vi "GenerateEventLog.vi"(0 "Instrument":string="Control", 2 "Check for file?":bool=TRUE) -> (3 "Global File Information":T1, 5 "File Path Out":path=path "D:/Data/2018-06-15/Proj_1/Temp Dependence/Control_200C.tdms")   [LabVIEW 2018]
uses:
  Global Variables.vi
  <vilib>/Utility/file.llb/Read Delimited Spreadsheet (string).vi
panel:
  in  "Path":path=path "E:/ProjectIndex.csv"
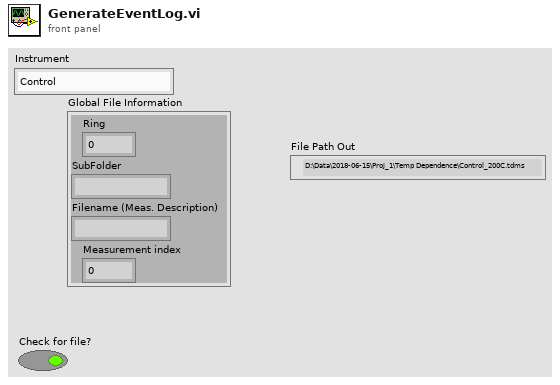
[diagram p1: front panel]
types:
  T1 = cluster{"Ring":u16, "SubFolder":string, "Filename (Meas. Description)":string, "Measurement index":i32}
  T2 = cluster{"Project":u16, "SubFolder":string, "Filename (Meas. Description)":string, "Measurement index":i32}
  T3 = cluster{"Project":u16, "SubFolder 2":string, "Meas. Description 2":string, "Measurement number 2":i32}
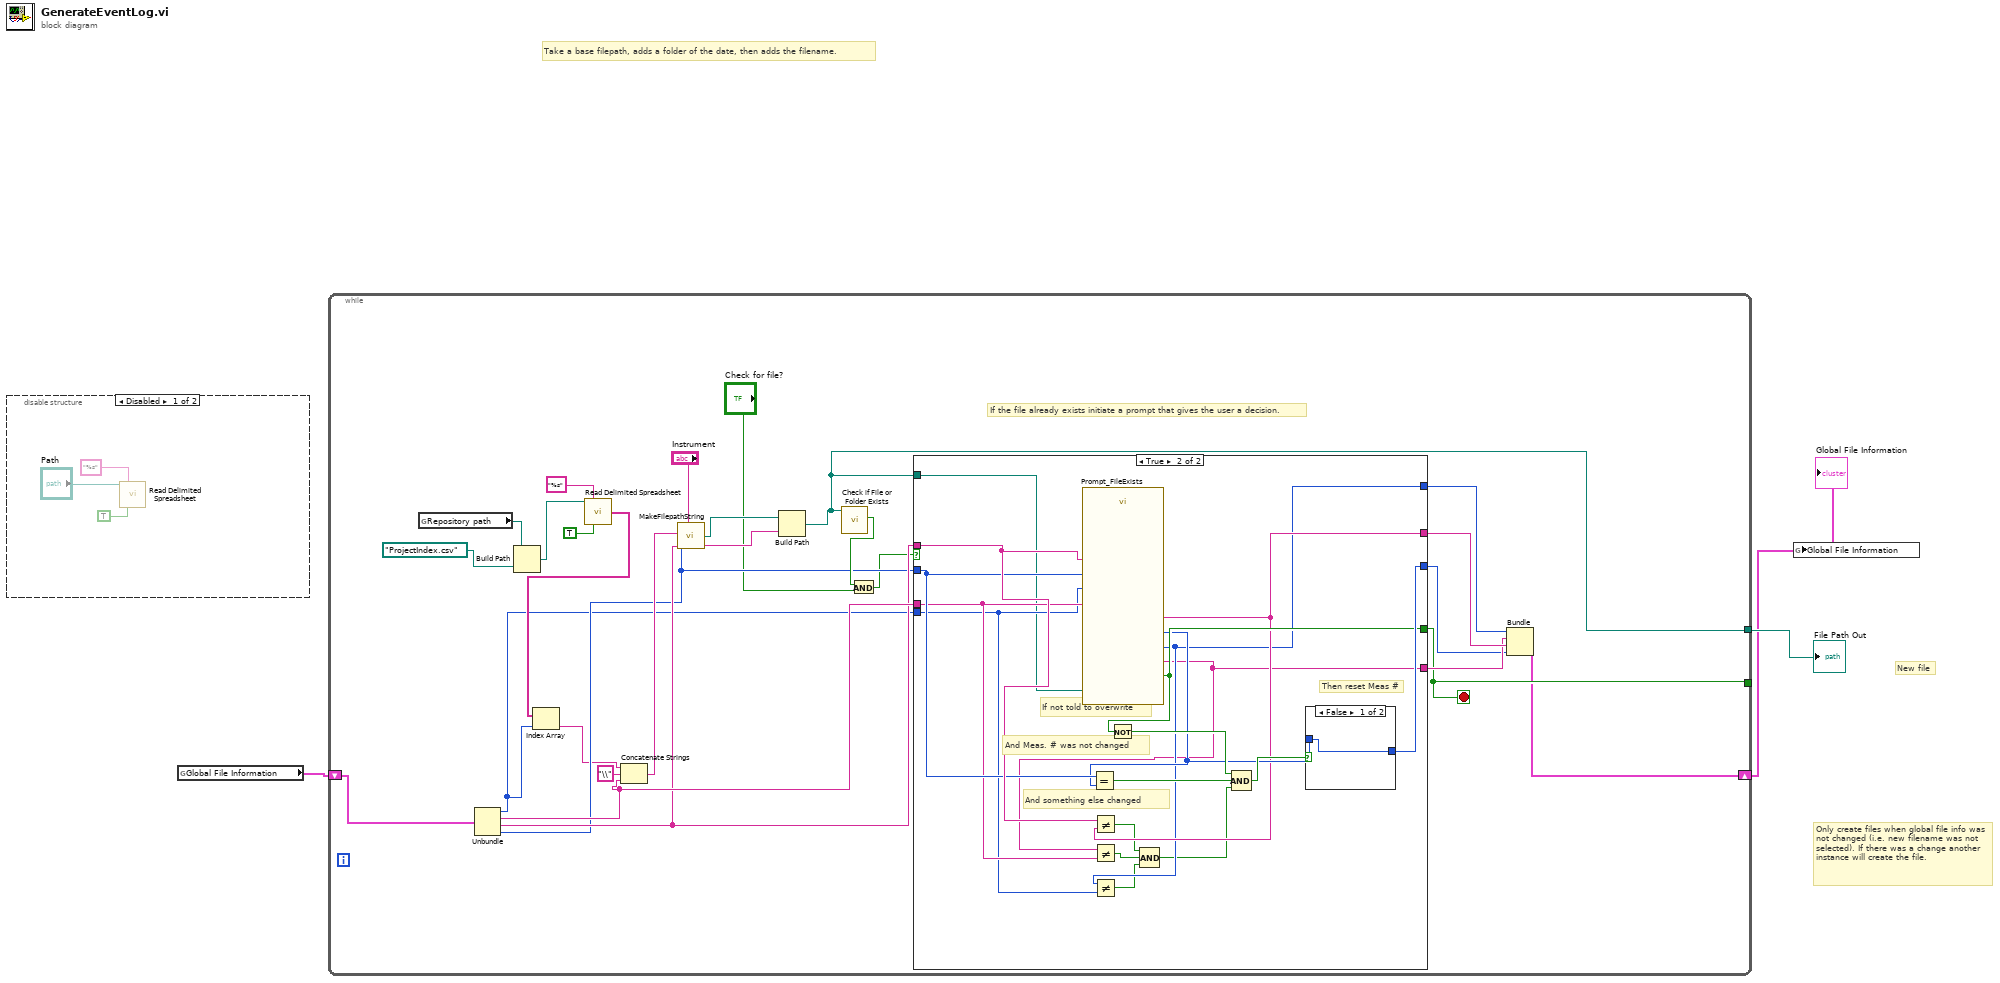
[diagram p0: block diagram]
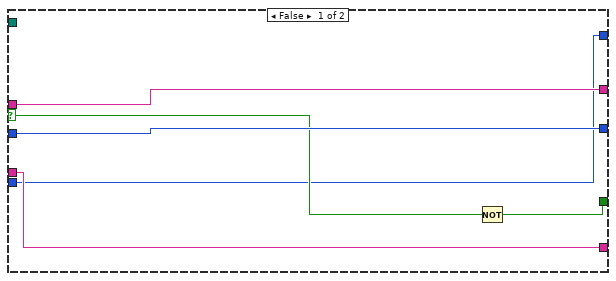
[diagram p3: hidden frame]
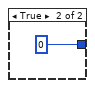
[diagram p4: hidden frame]
diagram:
  # "Only create files when global file info was not changed (i.e. new filename was not selected). If there was a change another instance will create the file."
  # "New file"
  # "Take a base filepath, adds a folder of the date, then adds the filename."
  n1 = disable-structure shown="Disabled" {
    frame Disabled {
      n2 = call-poly <vilib>:"Read Delimited Spreadsheet.vi"("file path (dialog if empty)"="Path", "format (%s)"="%s", "transpose? (F)"=TRUE) -> ("first row"=w4:string[])  [unwired: 7 in, 5 out]
    }
    frame Enabled {
    }
  }
  n3 = global read "Global Variables.vi" "Global File Information"() -> (w2:T2)
  n4 = while {
    tunnel: [w20] -> w3
    tunnel: [w19] -> _
    shift-right: [w17] -> w1
    shift-left: w2 -> [w16]
    stop <- w19 stop-if-true
    # "If the file already exists initiate a prompt that gives the user a decision."
    n5 = global read "Global Variables.vi" "Repository path"() -> (w15:path)
    n6 = Unbundle(w16) -> ("Project"=w9:u16, "SubFolder"=w29:string, "Filename (Meas. Description)"=w28:string, "Measurement index"=w27:i32)
    n7 = Build Path(base path=w15, name or relative path=path "ProjectIndex.csv" ("vi path")) -> (appended path=w14:path)
    n8 = call-poly <vilib>:"Read Delimited Spreadsheet.vi"("file path (dialog if empty)"=w14, "format (%s)"="%s", "transpose? (F)"=TRUE) -> ("first row"=w10:string[])  [unwired: 7 in, 5 out]
    n9 = Index Array(array=w10, index=w9) -> (element=w8:string)
    n10 = Concatenate Strings(w8, "\\" ("string"), w29) -> (w31:string)
    n11 = call "MakeFilepathString.vi"("Project"=w31, "Measurement number"=w27, "Extra"=w28, "Instrument"="Instrument") -> ("Folder"=w34:path, "Filename"=w33:string)  [unwired: 1 in, 1 out]
    n12 = Build Path(base path=w34, name or relative path=w33) -> (appended path=w20:path)
    n13 = call <vilib>:"Check if File or Folder Exists.vi"("path"=w20) -> ("file or folder exists?"=w30:bool)  [unwired: 8 in, 2 out]
    n14 = And(x=w30, y="Check for file?") -> (x .and. y?=w18:bool)
    n15 = case shown="True" w18 {
      selector: w18 -> [w38 _]
      tunnel: w27 -> [w40 w53]
      tunnel: w28 -> [w39 w54]
      tunnel: [w35 w46] -> w24
      tunnel: [w39 w50] -> w26
      tunnel: [w40 w58] -> w23
      tunnel: [w37 w52] -> w19
      tunnel: w9 -> [w35 w45]
      tunnel: w29 -> [w36 w49]
      tunnel: [w36 w42] -> w25
      tunnel: w20 -> [_ w41]
      frame False {
        n16 = Not(x=w38) -> (.not. x?=w37:bool)
      }
      frame True {
        # "Then reset Meas #"
        # "And something else changed"
        # "And Meas. # was not changed"
        # "If not told to overwrite"
        n17 = call "Prompt_FileExists.vi"("Attempted File Path"=w41, "Measurement number"=w53, "Meas. Description"=w54, "SubFolder"=w49, "Project"=w45) -> ("Overwrite"=w52:bool, "Meas. Description 2"=w50:string, "SubFolder 2"=w42:string, "Project 2"=w46:enum16{"H2TC", "VAPOR1"}, "Measurement number 2"=w51:i32)
        n18 = Equal?(x=w53, y=w51) -> (x = y?=w56:bool)
        n19 = Not Equal?(x=w54, y=w50) -> (x != y?=w48:bool)
        n20 = Not Equal?(x=w42, y=w49) -> (x != y?=w47:bool)
        n21 = Not Equal?(x=w46, y=w45) -> (x != y?=w44:bool)
        n22 = Not(x=w52) -> (.not. x?=w57:bool)
        n23 = Compound Arithmetic op=AND(w48, w47, w44) -> (w43:bool)
        n24 = Compound Arithmetic op=AND(w57, w56, w43) -> (w55:bool)
        n25 = case shown="False" w55 {
          tunnel: w51 -> [w59 _]
          tunnel: [w59 0] -> w58
          frame False {
          }
          frame True {
          }
        }
      }
    }
    n26 = Bundle("Project"=w24, "SubFolder 2"=w25, "Meas. Description 2"=w26, "Measurement number 2"=w23) -> (w17:T3)  [unwired: 1 in]
  }
  "File Path Out" <- w3
  "Global File Information" <- w1
  n27 = global write "Global Variables.vi" "Global File Information"(w1) -> ()
